vi "to_inline_table.vi"(8 "error in (no error)":errorcluster, 11 "Item in":refnum<class "Item.lvclass">) -> (0 "error out":errorcluster, 3 "InlineTable":refnum<class "InlineTable.lvclass">)   [LabVIEW 2020, in "toml_edit.lvlib" / "Item.lvclass"]
uses:
  Item.lvclass
  Item.lvclass/Item.ctl
  Value/Value.lvclass
  InlineTable/InlineTable.lvclass
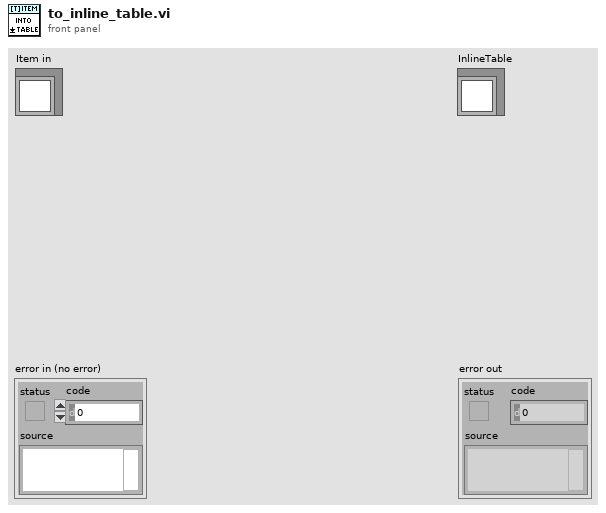
[diagram p1: front panel]
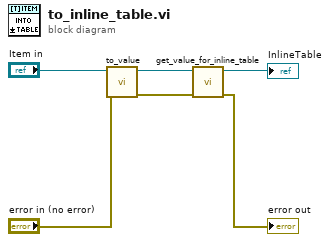
[diagram p0: block diagram]
diagram:
  n1 = call "to_value.vi"("error in (no error)"="error in (no error)", "Item in"="Item in") -> ("error out"=w5:errorcluster, "Value out"=w4:refnum<class "Value.lvclass">)  [unwired: 8 in]
  n2 = call "get_value_for_inline_table.vi"("error in (no error)"=w5, "Value in"=w4) -> ("error out"=→"error out":errorcluster, "InlineTable out"=→"InlineTable":refnum<class "InlineTable.lvclass">)  [unwired: 8 in]
